vi "Add Row.vi"(8 "error in (no error)":errorcluster, 11 "DataGrid in":refnum<class "DataGrid.lvclass">) -> (0 "error out":errorcluster, 3 "DataGrid out":refnum<class "DataGrid.lvclass">)   [LabVIEW 2018, in "DataGrid.lvclass"]
uses:
  DataGrid.lvclass
  C:/Program Files (x86)/National Instruments/LabVIEW 2018/vi.lib/QSI/QControls/QControl Classes/MulticolumnListbox/MulticolumnListbox.lvclass
  Read Configuration.vi
  <vilib>/QSI/DataGrid Configuration/DataGrid Config/DataGrid Config.lvclass
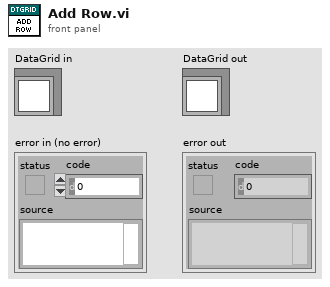
[diagram p1: front panel]
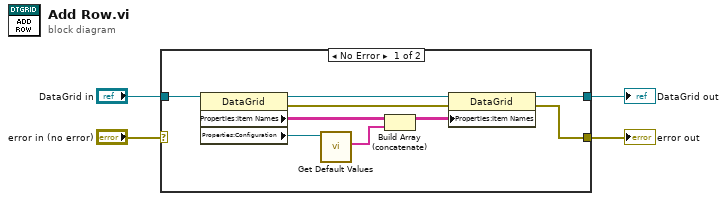
[diagram p0: block diagram]
diagram:
  n1 = case shown="No Error" "error in (no error)" {
    selector: "error in (no error)" -> [_ w15]
    tunnel: [w5 w15] -> w3
    tunnel: [w10 w14] -> w1
    tunnel: "DataGrid in" -> [w13 w14]
    frame No Error {
      n2 = property class="DataGrid"(reference=w13) -> (reference out=w12:refnum<class "DataGrid.lvclass">, error out=w6:errorcluster, "Properties:Item Names"=w9:string[][], "Properties:Configuration"=w11:refnum<class "DataGrid Config.lvclass">)  [unwired: 1 in]
      n3 = call <vilib>:"Get Default Values.vi"("DataGrid Config in"=w11) -> ("Default Values"=w8:string[])  [unwired: 8 in, 2 out]
      n4 = Build Array (concatenate)(w9, w8) -> (w7:string[][])
      n5 = property class="DataGrid"(reference=w12, error in=w6, "Properties:Item Names"=w7) -> (reference out=w10:refnum<class "DataGrid.lvclass">, error out=w5:errorcluster)
    }
    frame Error {
    }
  }
  "error out" <- w3
  "DataGrid out" <- w1
